vi "Stair_Case_Sequence.vi"() -> ()   [LabVIEW 2017]
uses:
  <vilib>/Analysis/1siggen.llb/Ramp Pattern by Delta.vi
  <vilib>/Utility/file.llb/Write To Spreadsheet File (DBL).vi
  <vilib>/Analysis/NI_AALBase.lvlib
  LabView_Automation/Keithley 6517/Keithley 6517.lvlib
panel:
  in  "file path (dialog if empty)":path
  in  "Sweep Start Voltage (1)":dbl=1.0
  in  "Ring":u16(ring) items=["Open and New"=3]
  in  "File Path Control":path
  out "Staircase Voltage":cluster{"Ramp Pattern":dbl[], dbl[]}(graph)
  in  "Sweep Bias Time (1 s)":dbl=1.0
  in  "Sweep Step Voltage (1)":dbl=1.0
  in  "Sweep Stop Voltage (10)":dbl=10.0
  in  "error in (no error)":errorcluster
  in  "VISA resource name":refnum<visa-resource-name>
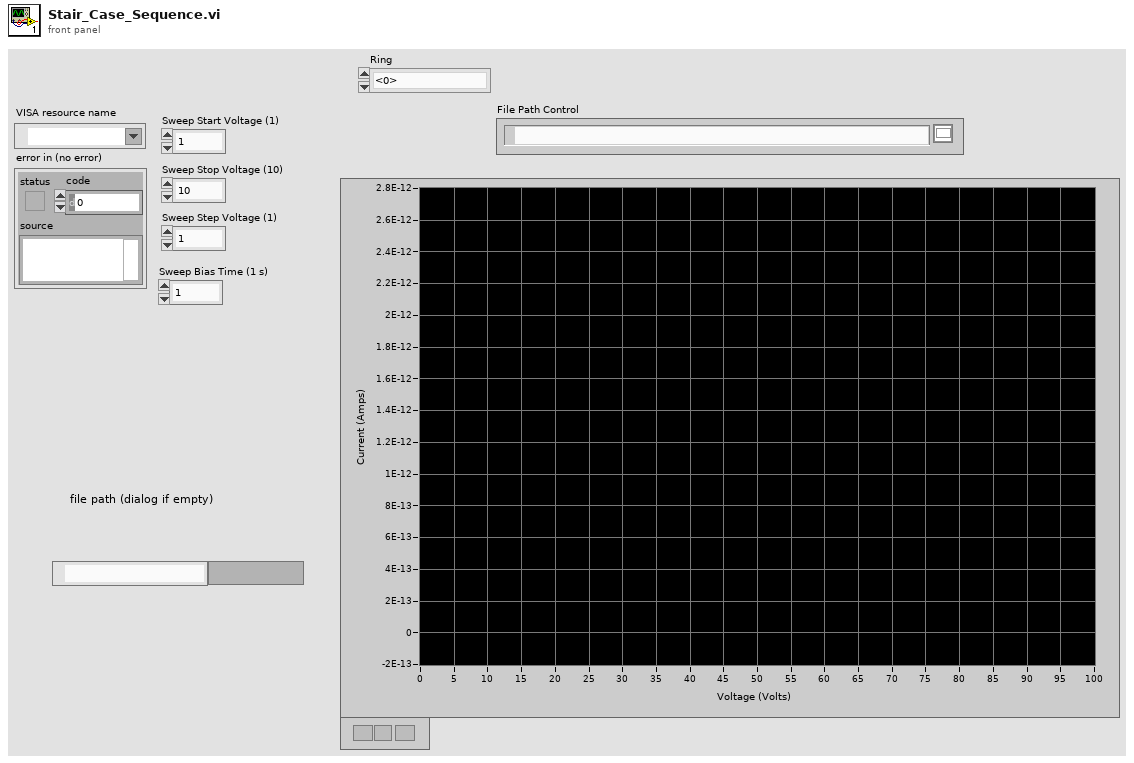
[diagram p1: front panel]
types:
  T1 = cluster{"Measurement":dbl, "Units":string, "Time Stamp and Date":string, "Reading #":dbl, "Channel #":dbl}
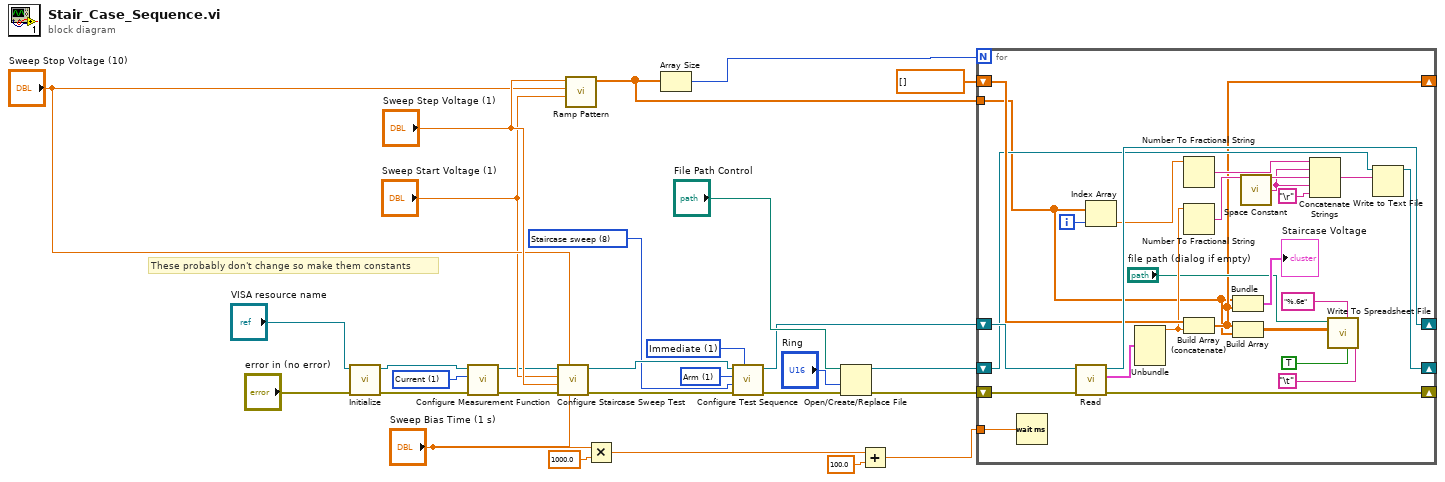
[diagram p0: block diagram]
diagram:
  w2 = 8 items=["Diode leakage", "Capacitor leakage", "Cable insulation resistance", "Resistor voltage coefficient", "Surface resistivity", "Volume resistivity", "Surface insulation resistance", "Square wave sweep", "Staircase sweep", "Alternating polarity resistance resistivity"] ("Test Sequence Type (9: Alternating polarity resistance resistivity)")
  w3 = 1 items=["Abort", "Arm"] ("Test Sequence Option (0: Abort)")
  w4 = 1 items=["Manual", "Immediate", "Bus", "External", "Trigger link", "Lid closure"] ("Control Source (0: Manual)")
  w25 = 1 items=["Voltage", "Current", "Resistance", "Charge"] ("Measurement Function (0: Voltage)")
  # "These probably don't change so make them constants"
  n1 = call "Initialize.vi"("error in (no error)"="error in (no error)", "VISA resource name"="VISA resource name") -> ("error out"=w26:errorcluster, "VISA resource name out"=w27:refnum<visa-resource-name>)  [unwired: 8 in]
  n2 = call "Configure Measurement Function.vi"("error in (no error)"=w26, "Measurement Function (0: Voltage)"=w25, "VISA resource name"=w27) -> ("error out"=w9:errorcluster, "VISA resource name out"=w10:refnum<visa-resource-name>)  [unwired: 7 in]
  n3 = call "Configure Staircase Sweep Test.vi"("Sweep Bias Time (1 s)"="Sweep Bias Time (1 s)", "Sweep Stop Voltage (10)"="Sweep Stop Voltage (10)", "error in (no error)"=w9, "Sweep Step Voltage (1)"="Sweep Step Voltage (1)", "Sweep Start Voltage (1)"="Sweep Start Voltage (1)", "VISA resource name"=w10) -> ("error out"=w7:errorcluster, "VISA resource name out"=w8:refnum<visa-resource-name>)  [unwired: 4 in]
  n4 = call-poly <vilib>:"Ramp Pattern.vi"("start"="Sweep Start Voltage (1)", "end"="Sweep Stop Voltage (10)", "delta"="Sweep Step Voltage (1)") -> ("Ramp Pattern"=w17:dbl[])  [unwired: 6 in, 2 out]
  n5 = Multiply(x="Sweep Bias Time (1 s)", y=1000.0) -> (x*y=w13:dbl)
  n6 = Array Size(array=w17) -> (size(s)=w1:i32)
  n7 = call "Configure Test Sequence.vi"("Control Source (0: Manual)"=w4, "error in (no error)"=w7, "Test Sequence Type (9: Alternating polarity resistance resistivity)"=w2, "Test Sequence Option (0: Abort)"=w3, "VISA resource name"=w8) -> ("error out"=w5:errorcluster, "VISA resource name out"=w6:refnum<visa-resource-name>)  [unwired: 5 in]
  n8 = Open/Create/Replace File(file path (use dialog)="File Path Control", error in=w5, access (0:read/write)="Ring") -> (refnum out=w21:refnum<file>, error out=w16:errorcluster)  [unwired: 3 in, 1 out]
  n9 = Add(x=w13, y=100.0) -> (x+y=w11:dbl)
  n10 = for {
    N: w1 -> [_]
    shift-right: [w52] -> _
    shift-left: w6 -> [w54]
    shift-right: [w51] -> _
    shift-left: w16 -> [w53]
    shift-right: [w31] -> _
    shift-left: dbl[] [] -> [w50]
    shift-right: [w42] -> _
    shift-left: w21 -> [w41]
    tunnel: w17 -> [w30]
    tunnel: w11 -> [w37]
    i -> [w38]
    n11 = Wait (ms)(milliseconds to wait=w37) -> ()  [unwired: 1 out]
    n12 = call "Read.vi"("error in (no error)"=w53, "VISA resource name"=w54) -> ("error out"=w51:errorcluster, "Measurement"=w48:T1, "VISA resource name out"=w52:refnum<visa-resource-name>)  [unwired: 7 in]
    n13 = Index Array(array=w30, index=w38) -> (element=w39:dbl)
    n14 = Unbundle(w48) -> ("Measurement"=w43:dbl)  [unwired: 4 out]
    n15 = Number To Fractional String(number=w39) -> (F-format string=w47:string)  [unwired: 3 in]
    n16 = Number To Fractional String(number=w43) -> (F-format string=w45:string)  [unwired: 3 in]
    n17 = Build Array (concatenate)(w50, w43) -> (w31:dbl[])
    n18 = Bundle("Ramp Pattern"=w30, w31) -> (→"Staircase Voltage":cluster{"Ramp Pattern":dbl[], dbl[]})  [unwired: 1 in]
    n19 = Build Array(w31, w30) -> (w36:dbl[][])
    n20 = call <vilib>:"Space Constant.vi"() -> ("String"=w40:string)
    n21 = Concatenate Strings(w47, w40, w45, w40, "\r") -> (w46:string)
    n22 = call-poly <vilib>:"Write To Spreadsheet File.vi"("delimiter (\\t)"="\t", "transpose? (no:F)"=TRUE, "format (%.3f)"="%.6e", "2D data"=w36, "file path (dialog if empty)"="file path (dialog if empty)") -> ()  [unwired: 3 in, 1 out]
    n23 = Write to Text File(file (use dialog)=w41, text=w46) -> (refnum out=w42:refnum<file>)  [unwired: 2 in, 2 out]
  }
